vi "Hi-Tec_Voltage_calculator.vi"(0 "Carrier_1 Q (l/min)":dbl=20.0 format="%.2f", 2 "Mode":enum16{"Control Hi-Tec", "Check Hi-Tec Demands"}(ring), 5 "Carrier_2 Q (l/min)":dbl=20.0 format="%.2f", 7 "Trace Q (l/min)":dbl=20.0 format="%.2f", 9 "Release temp (deg C)":dbl=20.0 format="%.2f", 11 "Atmos Pres (mbars)":dbl=1000.0 format="%.2f", 12 "Carrier Info":string) -> (4 "Carrier 1 Voltage":dbl format="%.3f", 6 "Carrier 2 Voltage":dbl format="%.2f", 8 "Trace Voltage":dbl format="%.2f", 10 "Flowrates (kg/min)":dbl[](array[numeric]) format="%.2f", 13 "Carrier 1_50 Voltage":dbl format="%.3f", 14 "Trace_2 Voltage":dbl format="%.2f", 15 "Error Comments":string)   [LabVIEW 2018]
uses:
  Anemometry/Anemometry Sub Vis/Globals/Gas_management_global.vi
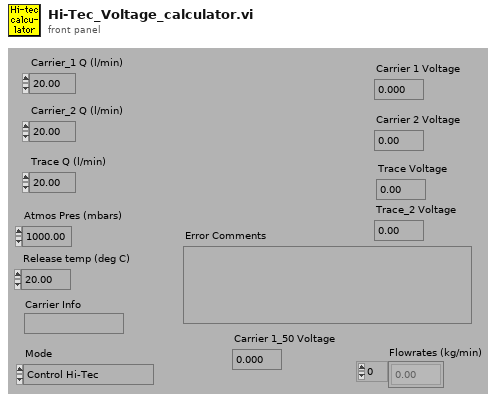
[diagram p1: front panel]
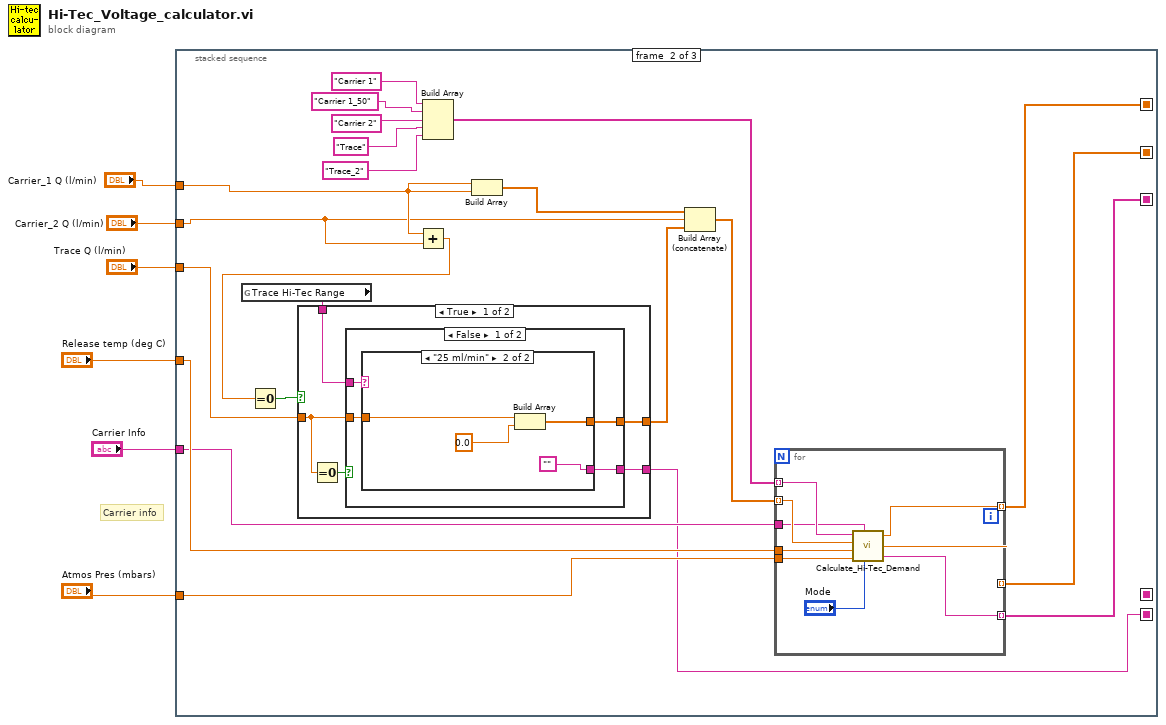
[diagram p0: block diagram]
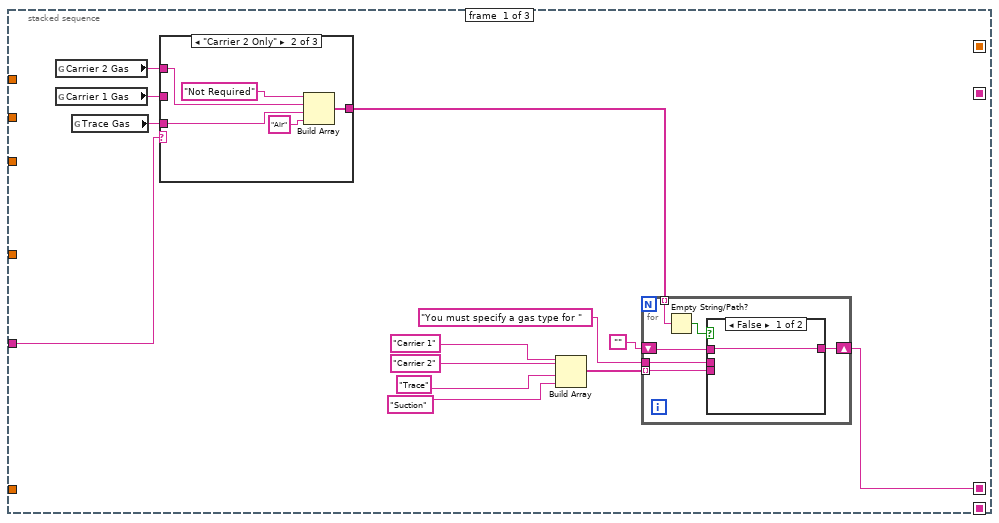
[diagram p2: hidden frame]
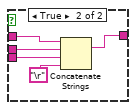
[diagram p3: hidden frame]
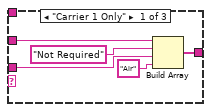
[diagram p4: hidden frame]
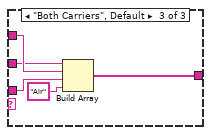
[diagram p5: hidden frame]
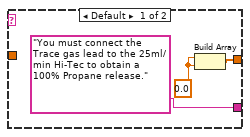
[diagram p6: hidden frame]
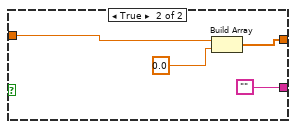
[diagram p7: hidden frame]
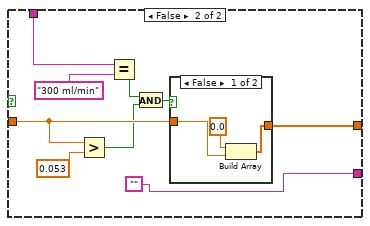
[diagram p8: hidden frame]
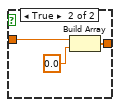
[diagram p9: hidden frame]
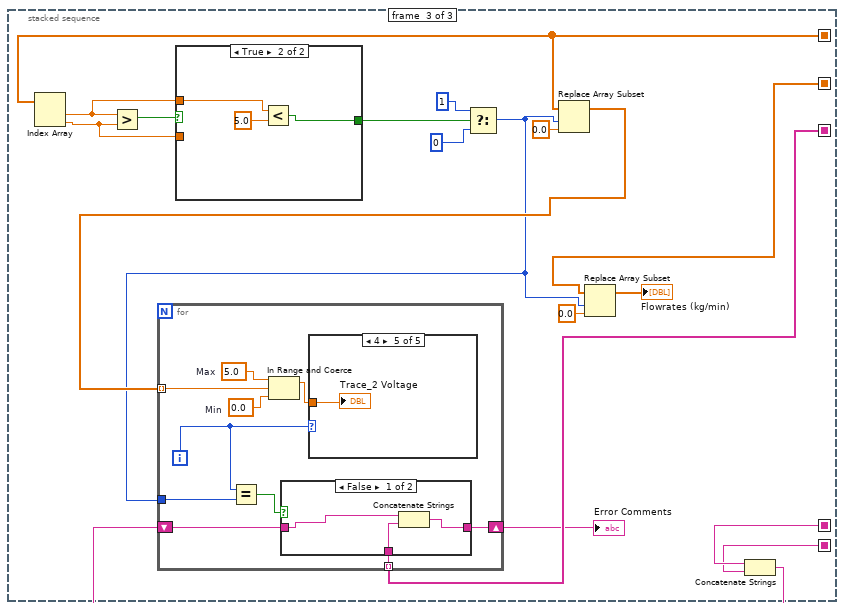
[diagram p10: hidden frame]
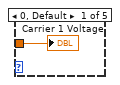
[diagram p12: hidden frame]
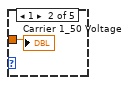
[diagram p13: hidden frame]
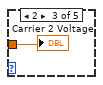
[diagram p14: hidden frame]
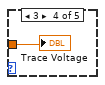
[diagram p15: hidden frame]
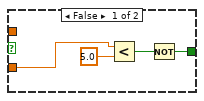
[diagram p16: hidden frame]
diagram:
  # "Carrier info"
  n1 = stacked-sequence {
    seq-local: [w9 _ _] -> [_ _ w115]
    seq-local: [_ w57 _] -> [_ _ w130]
    seq-local: [_ w56 _] -> [_ _ w121]
    seq-local: [_ w55 _] -> [_ _ w117]
    seq-local: [_ w48 _] -> [_ _ w114]
    tunnel: "Release temp (deg C)" -> [_ w67 _]
    tunnel: "Atmos Pres (mbars)" -> [_ w68 _]
    tunnel: "Carrier Info" -> [w7 w66 _]
    tunnel: "Trace Q (l/min)" -> [_ w50 _]
    tunnel: "Carrier_1 Q (l/min)" -> [_ w54 _]
    tunnel: "Carrier_2 Q (l/min)" -> [_ w53 _]
    frame #0 {
      n2 = global read "Gas_management_global.vi" "Carrier 2 Gas"() -> (w17:string)
      n3 = global read "Gas_management_global.vi" "Carrier 1 Gas"() -> (w19:string)
      n4 = global read "Gas_management_global.vi" "Trace Gas"() -> (w18:string)
      n5 = case shown="\"Carrier 2 Only\"" w7 {
        tunnel: [w34 w39 w45] -> w10
        tunnel: w19 -> [w33 _ w42]
        tunnel: w18 -> [w32 w37 w44]
        tunnel: w17 -> [_ w38 w43]
        frame "Carrier 1 Only" {
          n6 = Build Array(w33, "Not Required" ("Input Element"), w32, "Air") -> (w34:string[])
        }
        frame "Carrier 2 Only" {
          n7 = Build Array("Not Required" ("Input Element"), w38, w37, "Air") -> (w39:string[])
        }
        frame "Both Carriers", Default {
          n8 = Build Array(w42, w43, w44, "Air") -> (w45:string[])
        }
      }
      n9 = Build Array("Carrier 1" ("Gas Line Name"), "Carrier 2" ("Gas Line Name"), "Trace" ("Gas Line Name"), "Suction" ("Gas Line Name")) -> (w16:string[])
      n10 = for {
        shift-right: [w21] -> w9
        shift-left: "" -> [w22]
        tunnel: "You must specify a gas type for " -> [w24]
        tunnel: w16 -> [w23] mode=indexing
        tunnel: w10 -> [w20] mode=indexing
        n11 = Empty String/Path?(string/path=w20) -> (empty?=w25:bool)
        n12 = case shown="False" w25 {
          tunnel: w24 -> [_ w31]
          tunnel: w23 -> [_ w30]
          tunnel: w22 -> [w26 w29]
          tunnel: [w26 w28] -> w21
          frame False {
          }
          frame True {
            n13 = Concatenate Strings(w29, w31, w30, "\r") -> (w28:string)
          }
        }
      }
    }
    frame #1 {
      n14 = global read "Gas_management_global.vi" "Trace Hi-Tec Range"() -> (w49:string)
      n15 = Add(x=w54, y=w53) -> (x+y=w51:dbl)
      n16 = Equal To 0?(x=w51) -> (x = 0?=w47:bool)
      n17 = case shown="True" w47 {
        tunnel: [w73 w97] -> w52
        tunnel: w50 -> [w69 w96]
        tunnel: w49 -> [w72 w90]
        tunnel: [w71 ""] -> w48
        frame True {
          n18 = Equal To 0?(x=w69) -> (x = 0?=w70:bool)
          n19 = case shown="False" w70 {
            tunnel: [w77 w87] -> w73
            tunnel: w69 -> [w76 w85]
            tunnel: w72 -> [w75 _]
            tunnel: [w74 ""] -> w71
            frame False {
              n20 = case shown="\"25 ml/min\"" w75 {
                tunnel: [w79 w84] -> w77
                tunnel: w76 -> [_ w83]
                tunnel: ["You must connect the Trace gas lead to the 25ml/min Hi-Tec to obtain a 100% Propane release." ""] -> w74
                frame Default {
                  w80 = 0.0 ("element")
                  n21 = Build Array(w80, w80) -> (w79:dbl[])
                }
                frame "25 ml/min" {
                  n22 = Build Array(w83, 0.0 ("element")) -> (w84:dbl[])
                }
              }
            }
            frame True {
              n23 = Build Array(w85, 0.0 ("element")) -> (w87:dbl[])
            }
          }
        }
        frame False {
          n24 = Greater?(x=w96, y=0.053) -> (0:w91:bool)
          n25 = Equal?(x=w90, y="300 ml/min" ("Trace Hi-Tec Range")) -> (x = y?=w92:bool)
          n26 = And(x=w92, y=w91) -> (x .and. y?=w93:bool)
          n27 = case shown="False" w93 {
            tunnel: w96 -> [w99 w103]
            tunnel: [w100 w101] -> w97
            frame False {
              n28 = Build Array(0.0 ("element"), w99) -> (w100:dbl[])
            }
            frame True {
              n29 = Build Array(w103, 0.0 ("element")) -> (w101:dbl[])
            }
          }
        }
      }
      n30 = Build Array("Carrier 1" ("Gas Line Name"), "Carrier 1_50" ("Gas Line Name"), "Carrier 2" ("Gas Line Name"), "Trace" ("Gas Line Name"), "Trace_2" ("Gas Line Name")) -> (w64:string[])
      n31 = Build Array(w54, w54) -> (w58:dbl[])
      n32 = Build Array (concatenate)(w58, w53, w52) -> (w63:dbl[])
      n33 = for {
        tunnel: w68 -> [w112]
        tunnel: w67 -> [w111]
        tunnel: w63 -> [w110] mode=indexing
        tunnel: [w106] -> w56 mode=indexing
        tunnel: w64 -> [w109] mode=indexing
        tunnel: w66 -> [w107]
        tunnel: [w105] -> w57 mode=indexing
        tunnel: [w104] -> w55 mode=indexing
        n34 = call "Calculate_Hi-Tec_Demand.vi"("Gas Line Name"=w109, "Carrier Info"=w107, "Flowrate"=w110, "Release temp (deg C)"=w111, "Mode"="Mode", "Atmos Pres (mbars)"=w112) -> ("Demand Voltage"=w105:dbl, "Flowrate (kg/min)"=w106:dbl, "Error messages"=w104:string)
      }
    }
    frame #2 {
      n35 = Index Array(array=w130) -> (element #1=w124:dbl, element #2=w123:dbl)  [unwired: 2 in]
      n36 = Greater?(x=w124, y=w123) -> (0:w125:bool)
      n37 = case shown="True" w125 {
        tunnel: [w150 w156] -> w128
        tunnel: w124 -> [_ w154]
        tunnel: w123 -> [w152 _]
        frame False {
          n38 = Less?(x=w152, y=5.0) -> (x < y?=w151:bool)
          n39 = Not(x=w151) -> (.not. x?=w150:bool)
        }
        frame True {
          n40 = Less?(x=w154, y=5.0) -> (x < y?=w156:bool)
        }
      }
      n41 = Select(t=1 ("index"), s=w128, f=0 ("index")) -> (s? t:f=w118:i32)
      n42 = Replace Array Subset(array=w130, new element=0.0 ("new element/subarray"), index=w118) -> (w119:dbl[])
      n43 = Replace Array Subset(array=w121, new element=0.0 ("new element/subarray"), index=w118) -> (→"Flowrates (kg/min)":dbl[])
      n44 = Concatenate Strings(w115, w114) -> (w113:string)
      n45 = for {
        tunnel: w119 -> [w137] mode=indexing
        shift-right: [w133] -> w116
        shift-left: w113 -> [w132]
        tunnel: w118 -> [w135]
        tunnel: w117 -> [w131] mode=indexing
        i -> [w136]
        w139 = 0.0  # Min
        w138 = 5.0  # Max
        n46 = Equal?(x=w136, y=w135) -> (x = y?=w134:bool)
        n47 = In Range and Coerce(upper limit=w138, x=w137, lower limit=w139) -> (coerced(x)=w140:dbl)  [unwired: 1 out]
        n48 = case shown="False" w134 {
          tunnel: [w141 w144] -> w133
          tunnel: w132 -> [w143 w144]
          tunnel: w131 -> [w142 _]
          frame False {
            n49 = Concatenate Strings(w143, w142) -> (w141:string)
          }
          frame True {
          }
        }
        n50 = case shown="4" w136 {
          tunnel: w140 -> [w145 w146 w147 w148 w149]
          frame 0, Default {
            "Carrier 1 Voltage" <- w145
          }
          frame 1 {
            "Carrier 1_50 Voltage" <- w146
          }
          frame 2 {
            "Carrier 2 Voltage" <- w147
          }
          frame 3 {
            "Trace Voltage" <- w148
          }
          frame 4 {
            "Trace_2 Voltage" <- w149
          }
        }
      }
      "Error Comments" <- w116
    }
  }
